vi "Move Enum.vi"(6 "position":T1={"Left"=-1000, "Top"=-1000}, 7 "move?":bool, 8 "error in":errorcluster, 11 "Enum Array":refnum<vi>[](array[refnum])) -> (0 "error out":errorcluster)   [LabVIEW 2013, in "Table Manager.lvlib"]
uses:
  Table Manager.lvlib
  <vilib>/Utility/miscctls.llb/LVPositionTypeDef.ctl
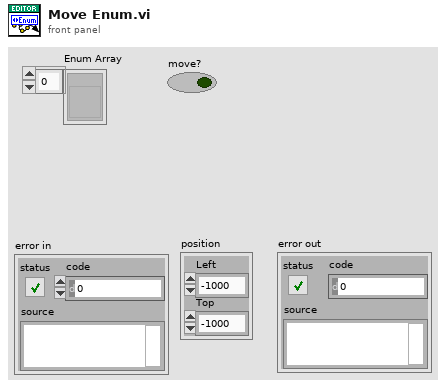
[diagram p1: front panel]
types:
  T1 = typedef "LVPositionTypeDef.ctl" = cluster{"Left":i32, "Top":i32}
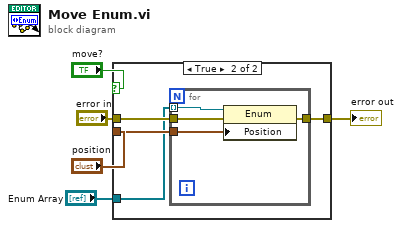
[diagram p0: block diagram]
diagram:
  n1 = case shown="True" "move?" {
    tunnel: "error in" -> [w6 w10]
    tunnel: [w6 w9] -> w5
    tunnel: "position" -> [_ w8]
    tunnel: "Enum Array" -> [_ w7]
    frame False {
    }
    frame True {
      n2 = for {
        tunnel: w10 -> [w14]
        tunnel: [w13] -> w9
        tunnel: w8 -> [w12]
        tunnel: w7 -> [w11] mode=indexing
        n3 = property on="Property Node" class="Enum"(reference=w11, error in=w14, "Position"=w12) -> (error out=w13:errorcluster)  [unwired: 1 out]
      }
    }
  }
  "error out" <- w5
